vi "Simple PID via Cryocon with ramp.vi"() -> ()   [LabVIEW 2016]
uses:
  <vilib>/addons/control/pid/pid.llb/PID (DBL).vi
  <vilib>/addons/control/pid/NI_PID_pid.lvlib
panel:
  in  "Ramp variable/second":dbl format="%#_13g"
  out "Setpoint":ext
  out "Elapsed Time (s)":dbl
  in  "milliseconds to wait":u32=500
  out "resulting string":string
  out "VISA Resource Name Out":refnum<visa-resource-name>
  out "error out":errorcluster
  in  "error in (no error)":errorcluster
  in  "CryoCon":refnum<visa-resource-name>
  in  "Stop":bool
  out "Process variable and Setpoint":cluster{"initial PV":dbl, "SP:":dbl}(graph)
  in  "PID gains":T1={"proportional gain (Kc)"=2.0, "integral time (Ti, min)"=2.0, "derivative time (Td, min)"=0.001} {"derivative time (Td, min)" format="%.3f"; "integral time (Ti, min)" format="%.3f"; "proportional gain (Kc)" format="%.3f"}
  out "PV:":dbl(slide)=60.754431603254424 scale=0.0..100.0
  in  "SP:":dbl(slide)=43000.0 min=0.0 max=0.0 scale=0.0..100.0
  out "MV:":dbl(slide)=18.78965245852964 scale=-100.0..100.0
  out "Manipulated variable":dbl(graph)
  in  "AH Bridge":refnum<visa-resource-name>
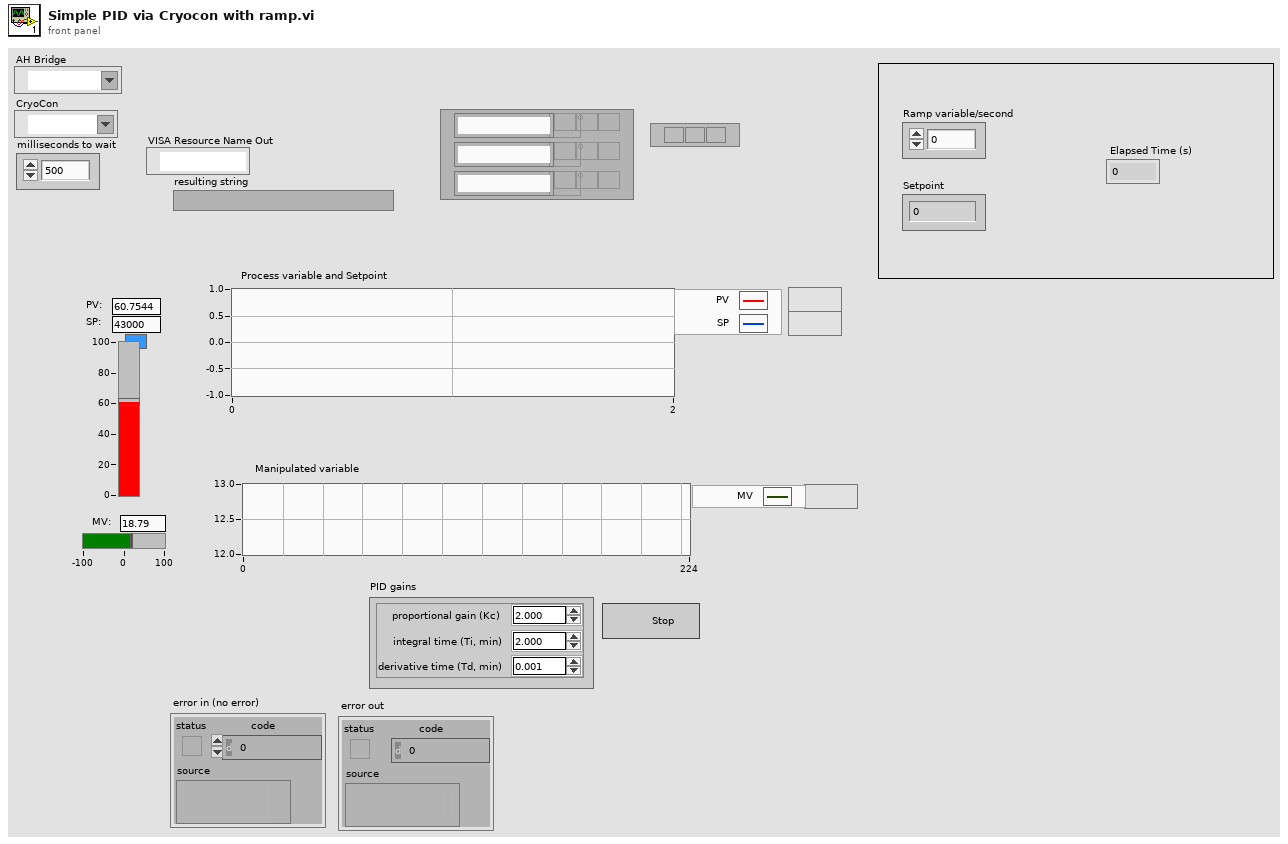
[diagram p1: front panel]
types:
  T1 = cluster{"proportional gain (Kc)":dbl, "integral time (Ti, min)":dbl, "derivative time (Td, min)":dbl}
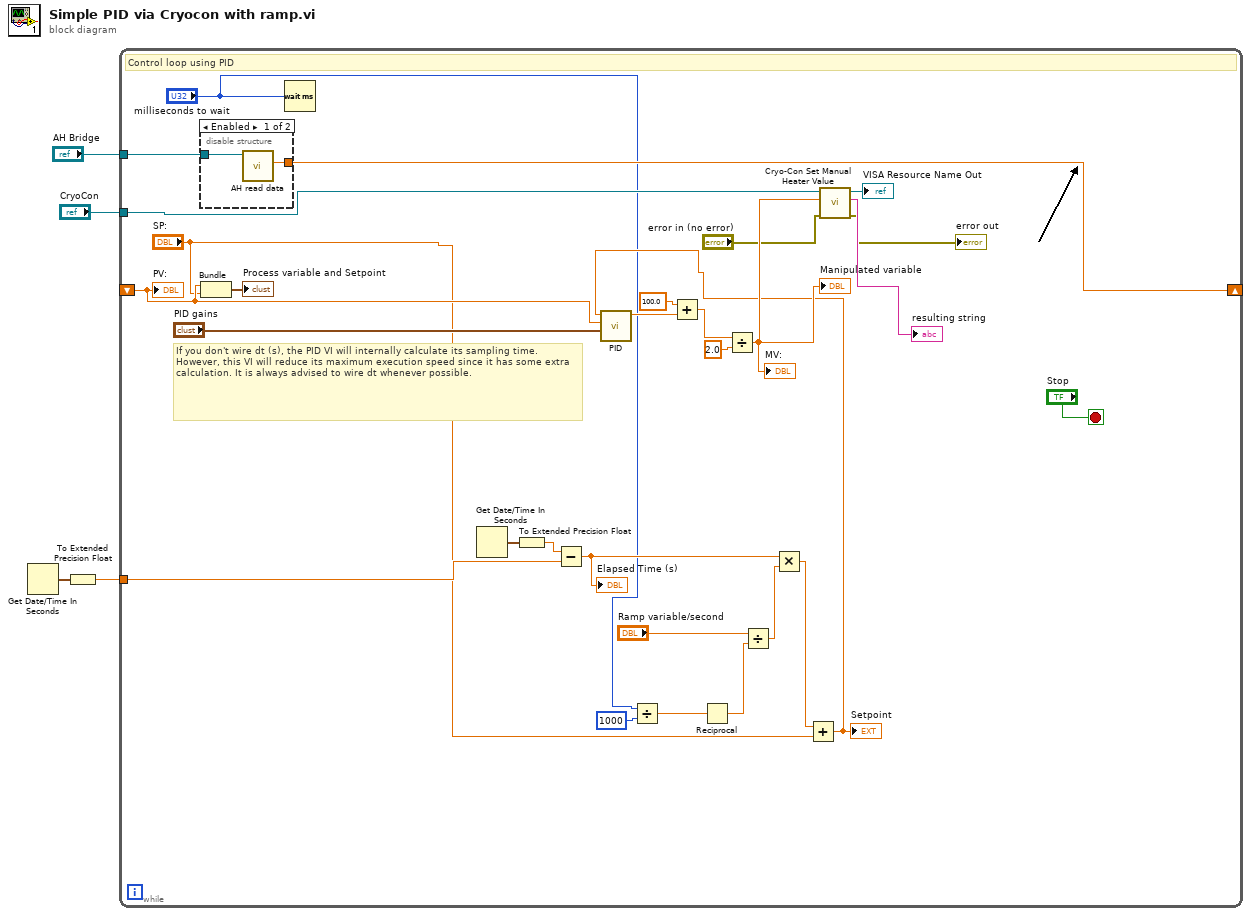
[diagram p0: block diagram]
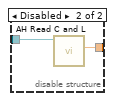
[diagram p2: hidden frame]
diagram:
  n1 = Get Date/Time In Seconds() -> (seconds since 1Jan1904=w2:timestamp)
  n2 = To Extended Precision Float(1:w2) -> (0:w1:ext)
  n3 = while {
    shift-left: _ -> [w31]
    shift-right: [w29] -> _
    tunnel: "AH Bridge" -> [w28]
    tunnel: "CryoCon" -> [w23]
    tunnel: w1 -> [w8]
    stop <- "Stop" stop-if-true
    # "If you don't wire dt (s), the PID VI will internally calculate its sampling time. However, this VI will reduce its maximum execution speed since it has some extra calculation. It is always advised to wire dt whenever possible."
    # "Control loop using PID"
    n4 = disable-structure shown="Enabled" {
      disable-tunnel: [w35 w36] -> w29
      disable-tunnel: w28 -> [w34 w37]
      frame Enabled {
        n5 = call "AH read data.vi"("VISA Resource Name"=w34) -> ("Capacitance"=w35:dbl)  [unwired: 7 in, 3 out]
      }
      frame Disabled {
        n6 = call "AH Read C and L.vi"("VISA resource name"=w37) -> ("Capacitance"=w36:dbl)  [unwired: 7 in, 3 out]
      }
    }
    n7 = Bundle("Capacitance"=w31, "SP:"="SP:") -> (→"Process variable and Setpoint":cluster{"Capacitance":dbl, "SP:":dbl})  [unwired: 1 in]
    n8 = Wait (ms)(milliseconds to wait="milliseconds to wait") -> ()  [unwired: 1 out]
    n9 = Get Date/Time In Seconds() -> (seconds since 1Jan1904=w17:timestamp)
    n10 = To Extended Precision Float(1:w17) -> (0:w16:ext)
    n11 = Subtract(x=w16, y=w8) -> (x-y=w15:ext)
    "Elapsed Time (s)" <- w15
    n12 = Divide(x="milliseconds to wait", y=u32 1000) -> (x/y=w11:dbl)
    n13 = Reciprocal(x=w11) -> (1/x=w12:dbl)
    n14 = Divide(x="Ramp variable/second", y=w12) -> (x/y=w13:dbl)
    n15 = Multiply(x=w15, y=w13) -> (x*y=w14:ext)
    n16 = Add(x=w14, y="SP:") -> (x+y=w6:ext)
    "Setpoint" <- w6
    n17 = call-poly <vilib>:"PID.vi"("PID gains"="PID gains", "process variable"=w31, "setpoint"=w6) -> ("output"=w27:dbl)  [unwired: 7 in, 1 out]
    n18 = Add(x=100.0, y=w27) -> (x+y=w25:dbl)
    n19 = Divide(x=w25, y=2.0) -> (x/y=w22:dbl)
    "MV:" <- w22
    "Manipulated variable" <- w22
    n20 = call "Cryo-Con Set Manual Heater Value.vi"("error in (no error)"="error in (no error)", "Set heat %"=w22, "VISA Resource Name"=w23) -> ("error out"=→"error out":errorcluster, "resulting string"=→"resulting string":string, "VISA Resource Name Out"=→"VISA Resource Name Out":refnum<visa-resource-name>)  [unwired: 6 in]
    "PV:" <- w31
  }
